vi "Get Winner.vi"(8 "error in (no error)":errorcluster, 11 "Match in":refnum<class "Match.lvclass">) -> (0 "error out":errorcluster, 2 "Winner":string, 3 "Match out":refnum<class "Match.lvclass">)   [LabVIEW 2016, in "Match.lvclass"]
uses:
  Match.lvclass
  Match.lvclass/Match.ctl
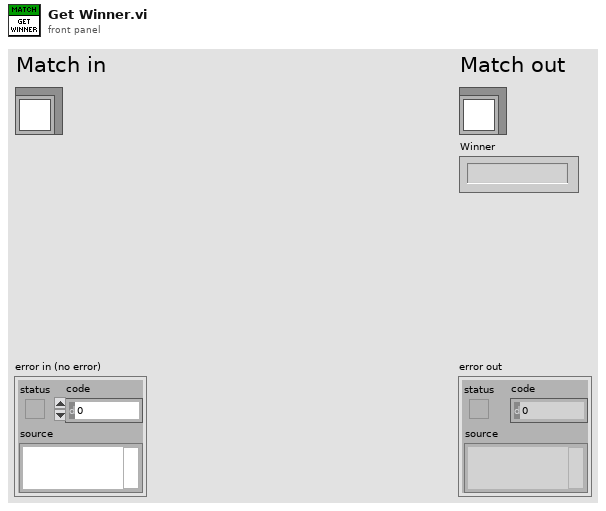
[diagram p1: front panel]
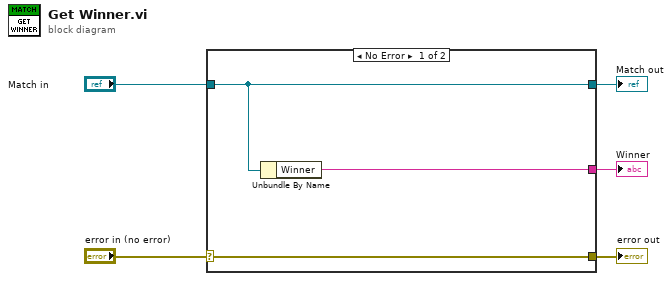
[diagram p0: block diagram]
diagram:
  n1 = case shown="No Error" "error in (no error)" {
    selector: "error in (no error)" -> [w8 w9]
    tunnel: [w8 w9] -> w4
    tunnel: [w7 w10] -> w2
    tunnel: "Match in" -> [w7 w10]
    tunnel: [w6 _] -> w1
    frame No Error {
      n2 = Unbundle By Name(w7) -> ("Winner"=w6:string)
    }
    frame Error {
    }
  }
  "error out" <- w4
  "Match out" <- w2
  "Winner" <- w1
